vi "配置文件read.vi"(8 "error in (no error)":errorcluster caption="错误输入（无错误）", 9 "configuration file path":path caption="配置文件的路径", 10 "键数组":string[](array[string]), 11 "段":string="应用程序交互") -> (0 "error out":errorcluster caption="错误输出", 2 "section exists?":bool caption="段存在？", 3 "updateconfiguration":T1={"主机"="27.154.58.30", "用户"="update", "密码"="std23506", "远程路径"="数据传输系统\\平台数据传输系统.exe", "下载文件名"="数据传输系统.exe", "软件版本"="V2.0.0.1"})   [LabVIEW 2016, in "数据传输系统-04.lvlib" / "update.lvlib"]
uses:
  <vilib>/Utility/config.llb/Read Key (I32).vi
  <vilib>/Utility/config.llb/Read Key (String).vi
  update.lvlib
  <vilib>/Utility/config.llb/NI_LVConfig.lvlib
  <vilib>/Utility/Data Type/NI_Data Type.lvlib
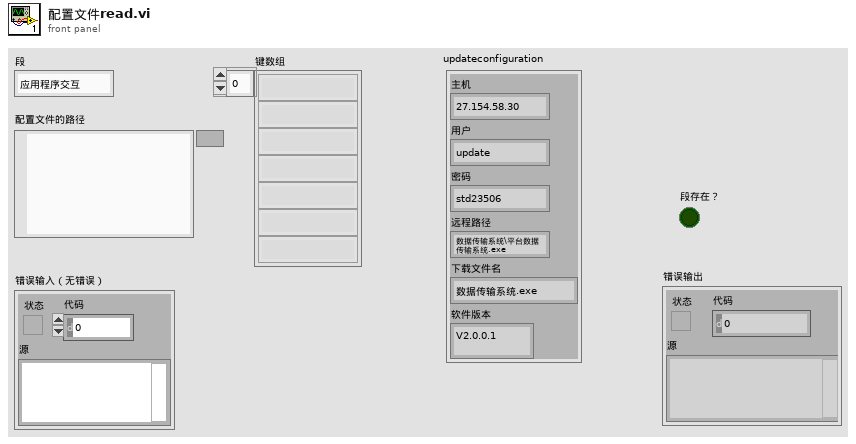
[diagram p1: front panel]
types:
  T1 = cluster{"主机":string, "用户":string, "密码":string, "远程路径":string, "下载文件名":string, "软件版本":string}
  T2 = typedef "NI_LVConfig.lvlib/Config Data RefNum.ctl" = refnum<k1>
  T3 = typedef "NI_Data Type.lvlib/Data Type.ctl" = enum8{"Invalid Type", "Void", "I8", "I16", "I32", "I64", "U8", "U16", "U32", "U64", "Single Float", "Double Float", "Extended Float", "Single Complex", "Double Complex", "Extended Complex", "Enum U8", "Enum U16", "Enum U32", "Enum U64", "Single Float With Unit", "Double Float With Unit", "Extended Float With Unit", "Single Complex with Unit", "Double Complex with Unit", "Extended Complex with Unit", "Boolean", "String", "Path", "Picture", "Tag", "Array", "Cluster", "Variant", "LV Variant", "Waveform", "Timestamp", "Digital Waveform", "Digital Data", "ExpressData", "Refnum", "External Data", "VI", "Poly VI", "LabVIEW Class Instance", "Fixed Point"}
  T4 = cluster{"[0]":string, "[1]":string, "[2]":string, "[3]":string, "[4]":string, "[5]":string}
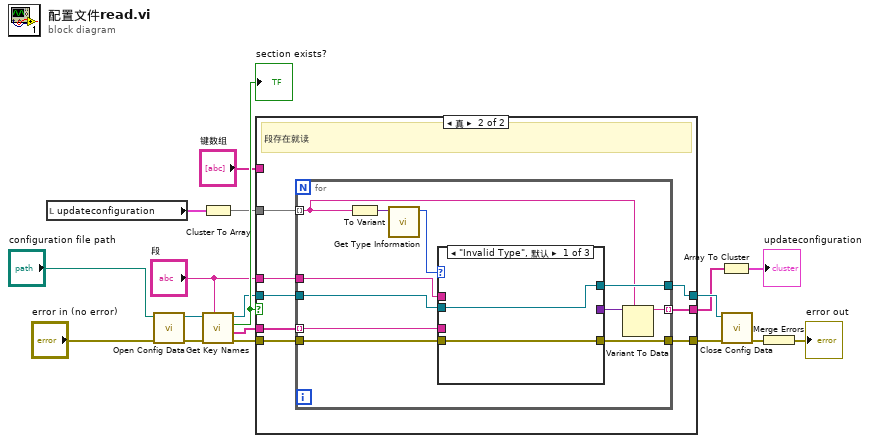
[diagram p0: block diagram]
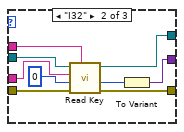
[diagram p3: hidden frame]
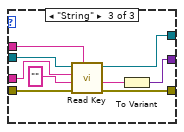
[diagram p4: hidden frame]
diagram:
  n1 = local read "updateconfiguration"() -> (w4:T1)
  n2 = call <vilib>:"Open Config Data.vi"("error in (no error)"="error in (no error)", "configuration file path"="configuration file path") -> ("error out"=w17:errorcluster, "refnum"=w18:T2)  [unwired: 7 in, 1 out]
  n3 = Cluster To Array(cluster=w4) -> (array=w3:string[])
  n4 = call <vilib>:"Get Key Names.vi"("section"="段", "error in (no error)"=w17, "refnum"=w18) -> ("error out"=w14:errorcluster, "key names"=w13:string[], "section exists?"=w16:bool, "refnum out"=w15:T2)  [unwired: 5 in]
  "section exists?" <- w16
  n5 = case shown="真" w16 {
    tunnel: w15 -> [w20 w27]
    tunnel: w14 -> [w19 w26]
    tunnel: w13 -> [_ w28]
    tunnel: "段" -> [_ w22]
    tunnel: [_ w25] -> w1
    tunnel: [w20 w24] -> w7
    tunnel: [w19 w23] -> w6
    tunnel: "键数组" -> [_ _]
    tunnel: w3 -> [_ w21]
    frame False {
      # "段不存在就赋初值"
    }
    frame True {
      # "段存在就读"
      n6 = for {
        tunnel: w28 -> [w35] mode=indexing
        tunnel: w27 -> [w37]
        tunnel: w26 -> [w34]
        tunnel: w22 -> [w38]
        tunnel: [w29] -> w25 mode=indexing
        tunnel: [w36] -> w24
        tunnel: [w33] -> w23
        tunnel: w21 -> [w30] mode=indexing
        n7 = To Variant(anything=w30) -> (Variant=w32:variant)
        n8 = call <vilib>:"Get Type Information.vi"("Variant"=w32) -> ("Type"=w39:T3)  [unwired: 6 in, 4 out]
        n9 = case shown="\"Invalid Type\", 默认" w39 {
          tunnel: w38 -> [_ w49 w58]
          tunnel: w37 -> [w41 w47 w57]
          tunnel: [w41 w46 w56] -> w36
          tunnel: w35 -> [_ w48 w55]
          tunnel: w34 -> [w40 w44 w54]
          tunnel: [w40 w43 w53] -> w33
          tunnel: [_ w42 w51] -> w31
          frame "Invalid Type", Default {
          }
          frame "I32" {
            n10 = call-poly <vilib>:"Read Key.vi"("section"=w49, "error in (no error)"=w44, "default value"=0, "key"=w48, "refnum"=w47) -> ("error out"=w43:errorcluster, "value"=w45:i32, "refnum out"=w46:T2)  [unwired: 3 in, 1 out]
            n11 = To Variant(anything=w45) -> (Variant=w42:variant)
          }
          frame "String" {
            n12 = call-poly <vilib>:"Read Key.vi"("section"=w58, "error in (no error)"=w54, "default value"="", "key"=w55, "refnum"=w57) -> ("error out"=w53:errorcluster, "value"=w52:string, "refnum out"=w56:T2)  [unwired: 3 in, 1 out]
            n13 = To Variant(anything=w52) -> (Variant=w51:variant)
          }
        }
        n14 = Variant To Data(type=w30, Variant=w31) -> (data=w29:string)  [unwired: 1 in, 1 out]
      }
    }
  }
  n15 = Array To Cluster(array=w1) -> (cluster=→"updateconfiguration":T4)
  n16 = call <vilib>:"Close Config Data.vi"("error in (no error)"=w6, "refnum"=w7) -> ("error out"=w11:errorcluster)  [unwired: 8 in, 1 out]
  n17 = Merge Errors(w11) -> (→"error out":errorcluster)
